vi "Update Objective calibration data.vi"(8 "error in (no error)":errorcluster, 9 "System Config":T1={"Laser wavelength (nm)"=920.0, "DAQ FPGA System"={"Clock Freq (MHz) "=200.0, "Samples Wait after Trigger"=5080, "AOD fill"=4900, "StartupDelay"=0, "Slip Cycle (clock cycles)"=600000, "Add Cycle"=TRUE}, "Control system"={"AOD 1 Amplitude"=0, "AOD 2 Amplitude"=0, "AOD 3 Amplitude"=0, "AOD 4 Amplitude"=0, "AOD 5 Amplitude"=0, "AOD 6 Amplitude"=0, "T0 (ns)"=0.0, "Ta (ns)"=0.0, "Data Time Interval (ns)"=0.0, "Ctrl FPGA Clock (MHz)"=240.0}} {"Control system"."Ctrl FPGA Clock (MHz)" min=80.0 max=500.0 step=1.0; "Control system"."Data Time Interval (ns)" min=0.0 max=2048.0 step=1.0; "Control system"."Ta (ns)" min=0.0 max=2048.0 step=1.0; "Control system"."T0 (ns)" min=0.0 max=2048.0 step=1.0; "Control system"."AOD 6 Amplitude" min=0 max=2048 step=1; "Control system"."AOD 5 Amplitude" min=0 max=2048 step=1; "Control system"."AOD 4 Amplitude" min=0 max=2048 step=1; "Control system"."AOD 3 Amplitude" min=0 max=2048 step=1; "Control system"."AOD 2 Amplitude" min=0 max=2048 step=1; "Control system"."AOD 1 Amplitude" min=0 max=2048 step=1; "Laser wavelength (nm)" min=800.0 max=1080.0 step=1.0}, 10 "Config cluster OUT":T5, 11 "Current Calibration Parameters in":T4) -> (0 "error out":errorcluster, 3 "Current Calibration Parameters out":T4)   [LabVIEW 2020]
uses:
  TypeDefs/Current Calibration Parameters.ctl
  Typedefs/Calibration config.ctl
  Typedefs/Objective Config.ctl
  Typedefs/Prechirper Cal Config.ctl
  Typedefs/PreChirper constants.ctl
  Typedefs/System Configuration.ctl
  Typedefs/DAQ FPGA system config.ctl
  Typedefs/CTRL system config.ctl
  Globals/gl_Calibration globals.vi
panel:
  in  "Use FP objectives":bool
  in  "Current Objective":string
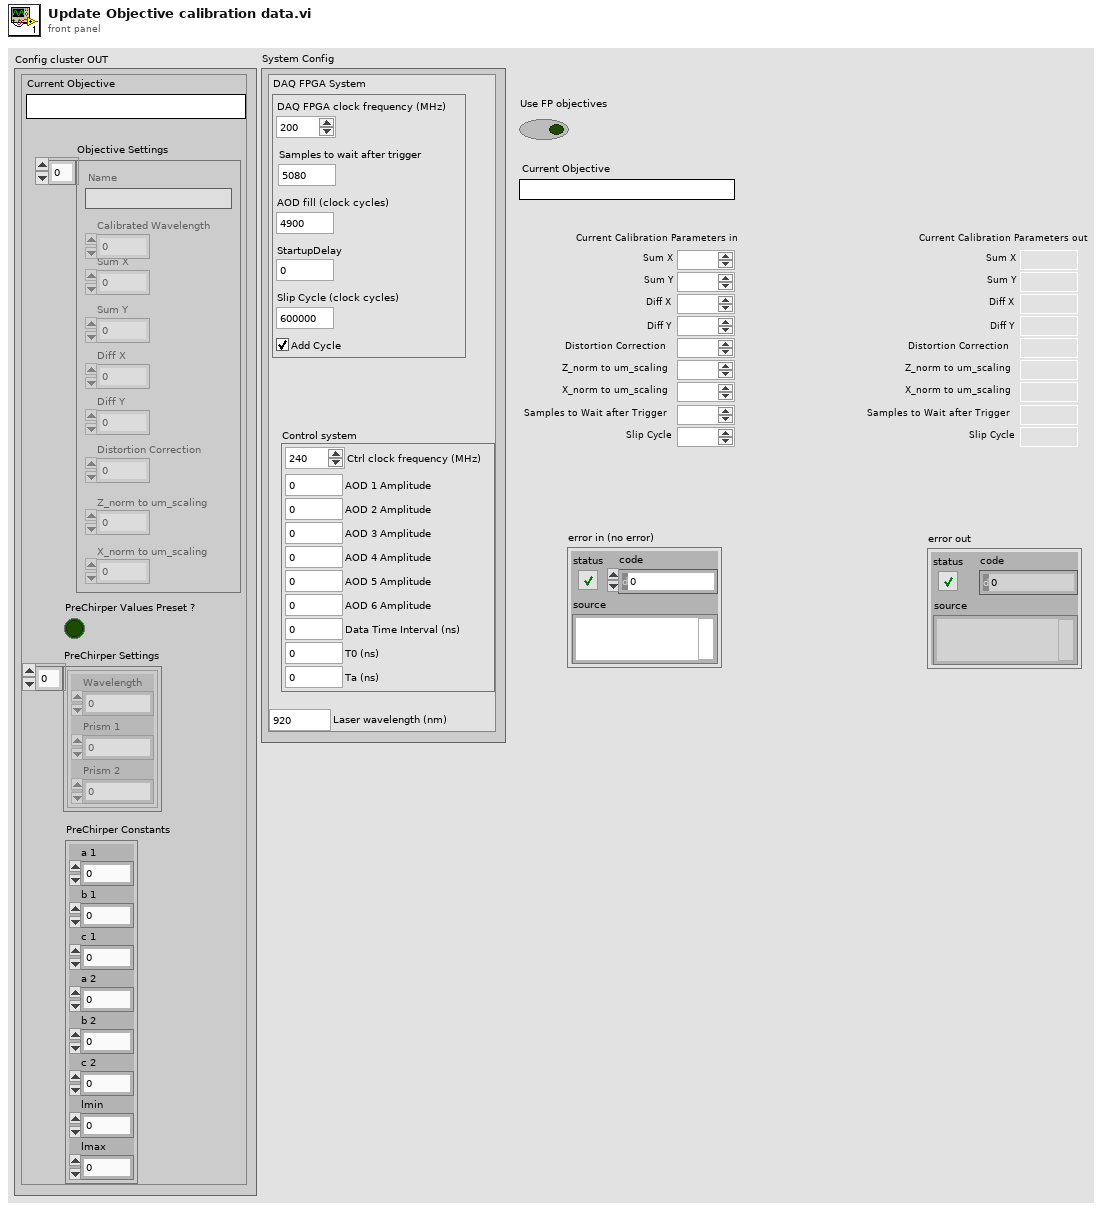
[diagram p1: front panel]
types:
  T1 = typedef "System Configuration.ctl" = cluster{"Laser wavelength (nm)":dbl, "DAQ FPGA System":T2, "Control system":T3}
  T2 = typedef "DAQ FPGA system config.ctl" = cluster{"Clock Freq (MHz) ":dbl, "Samples Wait after Trigger":u16, "AOD fill":u16, "StartupDelay":i32, "Slip Cycle (clock cycles)":u32, "Add Cycle":bool}
  T3 = typedef "CTRL system config.ctl" = cluster{"AOD 1 Amplitude":i16, "AOD 2 Amplitude":i16, "AOD 3 Amplitude":i16, "AOD 4 Amplitude":i16, "AOD 5 Amplitude":i16, "AOD 6 Amplitude":i16, "T0 (ns)":dbl, "Ta (ns)":dbl, "Data Time Interval (ns)":dbl, "Ctrl FPGA Clock (MHz)":dbl}
  T4 = typedef "Current Calibration Parameters.ctl" = cluster{"Sum X":dbl, "Sum Y":dbl, "Diff X":dbl, "Diff Y":dbl, "Distortion Correction":dbl, "Z_norm to um_scaling":dbl, "X_norm to um_scaling":dbl, "Samples to Wait after Trigger":dbl, "Slip Cycle":dbl}
  T5 = typedef "Calibration config.ctl" = cluster{"Current Objective":string, "Objective Settings":T6[], "PreChirper Values Preset ?":bool, "PreChirper Settings":T7[], "PreChirper Constants":T8}
  T6 = typedef "Objective Config.ctl" = cluster{"Name":string, "Sum X":dbl, "Sum Y":dbl, "Diff X":dbl, "Diff Y":dbl, "Distortion Correction":dbl, "Z_norm to um_scaling":dbl, "X_norm to um_scaling":dbl, "Calibrated Wavelength":dbl}
  T7 = typedef "Prechirper Cal Config.ctl" = cluster{"Wavelength":i32, "Prism 1":i32, "Prism 2":i32}
  T8 = typedef "PreChirper constants.ctl" = cluster{"a 1":i32, "b 1":i32, "c 1":i32, "a 2":i32, "b 2":i32, "c 2":i32, "lmin":i32, "lmax":i32}
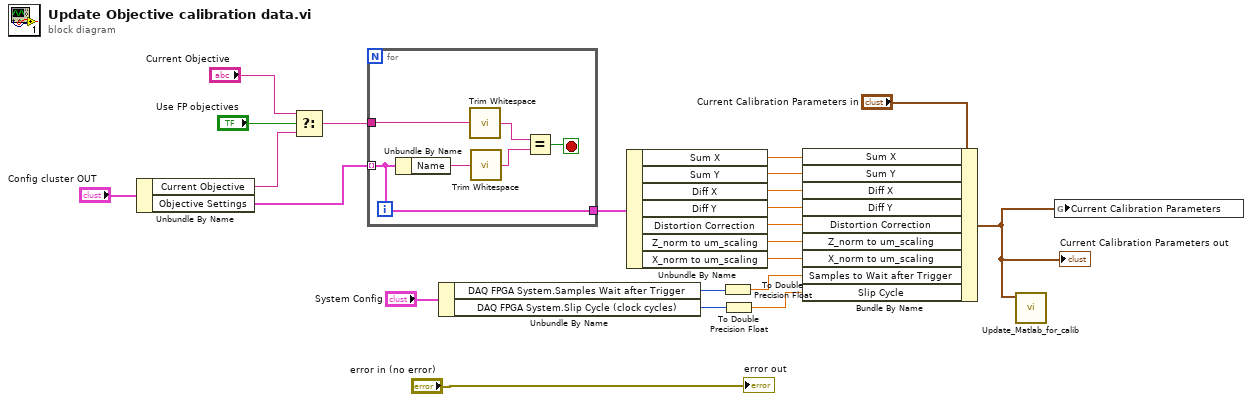
[diagram p0: block diagram]
diagram:
  n1 = Unbundle By Name("Config cluster OUT") -> ("Current Objective"=w19:string, "Objective Settings"=w16:T6[])
  n2 = Select(t="Current Objective", s="Use FP objectives", f=w19) -> (s? t:f=w18:string)
  n3 = for {
    tunnel: w18 -> [w27]
    tunnel: w16 -> [w23] mode=indexing
    tunnel: [w23] -> w15
    stop <- w24 stop-if-true
    n4 = Unbundle By Name(w23) -> ("Name"=w28:string)
    n5 = call <vilib>:"Trim Whitespace.vi"("string"=w27) -> ("trimmed string"=w26:string)  [unwired: 1 in]
    n6 = call <vilib>:"Trim Whitespace.vi"("string"=w28) -> ("trimmed string"=w25:string)  [unwired: 1 in]
    n7 = Equal?(x=w26, y=w25) -> (x = y?=w24:bool)
  }
  n8 = Unbundle By Name("System Config") -> ("DAQ FPGA System.Samples Wait after Trigger"=w5:u16, "DAQ FPGA System.Slip Cycle (clock cycles)"=w4:u32)
  n9 = Unbundle By Name(w15) -> ("Sum X"=w14:dbl, "Sum Y"=w13:dbl, "Diff X"=w12:dbl, "Diff Y"=w11:dbl, "Distortion Correction"=w10:dbl, "Z_norm to um_scaling"=w9:dbl, "X_norm to um_scaling"=w8:dbl)
  n10 = To Double Precision Float(number=w5) -> (double precision float=w3:dbl)
  n11 = To Double Precision Float(number=w4) -> (double precision float=w2:dbl)
  n12 = Bundle By Name(cluster="Current Calibration Parameters in", "Sum X"=w14, "Sum Y"=w13, "Diff X"=w12, "Diff Y"=w11, "Distortion Correction"=w10, "Z_norm to um_scaling"=w9, "X_norm to um_scaling"=w8, "Samples to Wait after Trigger"=w3, "Slip Cycle"=w2) -> (w1:T4)
  "Current Calibration Parameters out" <- w1
  n13 = call "Update_Matlab_for_calib.vi"("Current Calibration Parameters"=w1) -> ()  [unwired: 10 in, 1 out]
  n14 = global write "gl_Calibration globals.vi" "Current Calibration Parameters"(w1) -> ()
  "error out" <- "error in (no error)"
